vi "Fire DIStateChanged Event_DAQ.vi"(4 "Falling":bool, 6 "Rising":bool, 7 "FireEvTrigger":T1, 8 "error in (no error)":errorcluster, 10 "Name":string, 11 "DIStateChangeEv":refnum<user-event>) -> (0 "error out":errorcluster)   [LabVIEW 2022 SP3, in "DAQ.lvclass"]
doc: "Developed by Kevin Thompson\nkevin@thompsonengineering.net\n\nCopyright 2018-2020\nThompson Engineering, LLC"
uses:
  DAQ.lvclass
  DataTypes/TD DAQ DI state change ev.ctl
  DataTypes/TD FireDIStateChangeEventTrigger--cluster.ctl
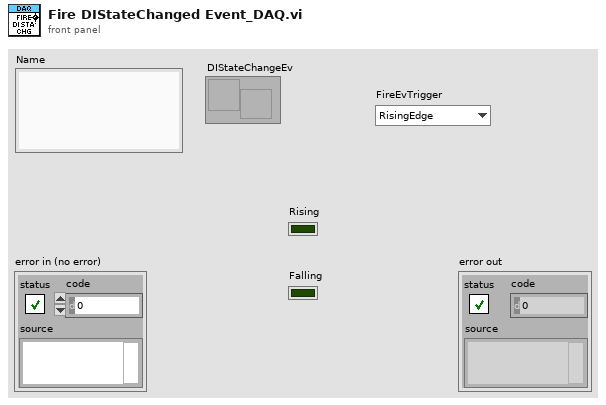
[diagram p1: front panel]
types:
  T1 = typedef "TD FireDIStateChangeEventTrigger--cluster.ctl" = enum16{"RisingEdge", "FallingEdge", "Both", "Disable"}
  T2 = typedef "TD DAQ DI state change ev.ctl" = cluster{"Time Stamp":timestamp, "Name":string, "vData":variant}
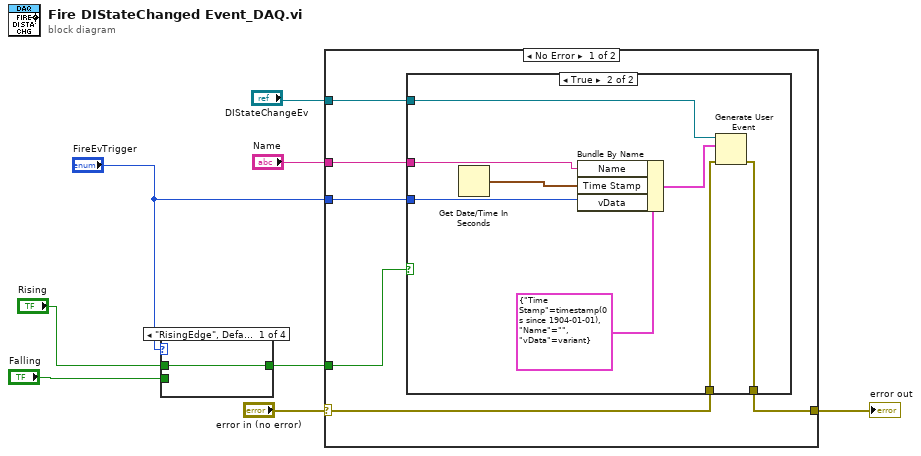
[diagram p0: block diagram]
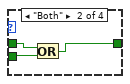
[diagram p2: hidden frame]
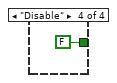
[diagram p4: hidden frame]
diagram:
  n1 = case shown="\"RisingEdge\", Default" "FireEvTrigger" {
    tunnel: "Falling" -> [_ w11 w13 _]
    tunnel: [w9 w10 w13 FALSE ("Falling")] -> w2
    tunnel: "Rising" -> [w9 w12 _ _]
    frame "RisingEdge", Default {
    }
    frame "Both" {
      n2 = Or(x=w12, y=w11) -> (x .or. y?=w10:bool)
    }
    frame "FallingEdge" {
    }
    frame "Disable" {
    }
  }
  n3 = case shown="No Error" "error in (no error)" {
    selector: "error in (no error)" -> [w19 w30]
    tunnel: [w20 w30] -> w7
    tunnel: "Name" -> [w18 _]
    tunnel: "DIStateChangeEv" -> [w17 _]
    tunnel: "FireEvTrigger" -> [w16 _]
    tunnel: w2 -> [w15 _]
    frame No Error {
      n4 = case shown="True" w15 {
        tunnel: [w21 w29] -> w20
        tunnel: w19 -> [w21 w28]
        tunnel: w18 -> [_ w27]
        tunnel: w17 -> [_ w26]
        tunnel: w16 -> [_ w25]
        frame False {
        }
        frame True {
          n5 = Get Date/Time In Seconds() -> (seconds since 1Jan1904=w24:timestamp)
          n6 = Bundle By Name(cluster=T2 {"Time Stamp"=timestamp(0 s since 1904-01-01), "Name"="", "vData"=variant} ("event data"), "Name"=w27, "Time Stamp"=w24, "vData"=w25) -> (w22:T2)
          n7 = Generate User Event(user event=w26, event data cluster=w22, error in=w28) -> (error out=w29:errorcluster)  [unwired: 1 in, 1 out]
        }
      }
    }
    frame Error {
    }
  }
  "error out" <- w7
